vi "example_04_make_installer.vi"() -> ()   [LabVIEW 2015, in "lv-bin-7zip.lvlib" / "v1.lvlib"]
uses:
  v1.lvlib
  <userlib>/antonio-alexander/lv-bin/lv-bin/public/api/v1/advanced/add_data_path_multiple.vi
  advanced/make_installer_exe_simple.vi
  <userlib>/antonio-alexander/lv-bin/lv-bin/public/api/v1/v1.lvlib
  lv-bin-7zip.lvlib
panel:
  out "temp_folder (deleted)":path
  in  "bin_path":path
  out "setup_filename out":path
  out "error out":errorcluster
  in  "setup_filename in":path
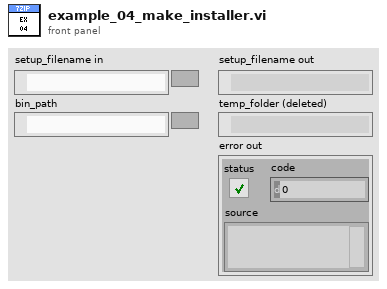
[diagram p1: front panel]
types:
  T1 = enum16{"open", "replace", "create", "open or create", "replace or create", "replace or create with confirmation"}
  T2 = typedef "lv-bin.lvlib/v1.lvlib/temp_dir_config.ctl" = cluster{"root_folder":path, "prefix":string}
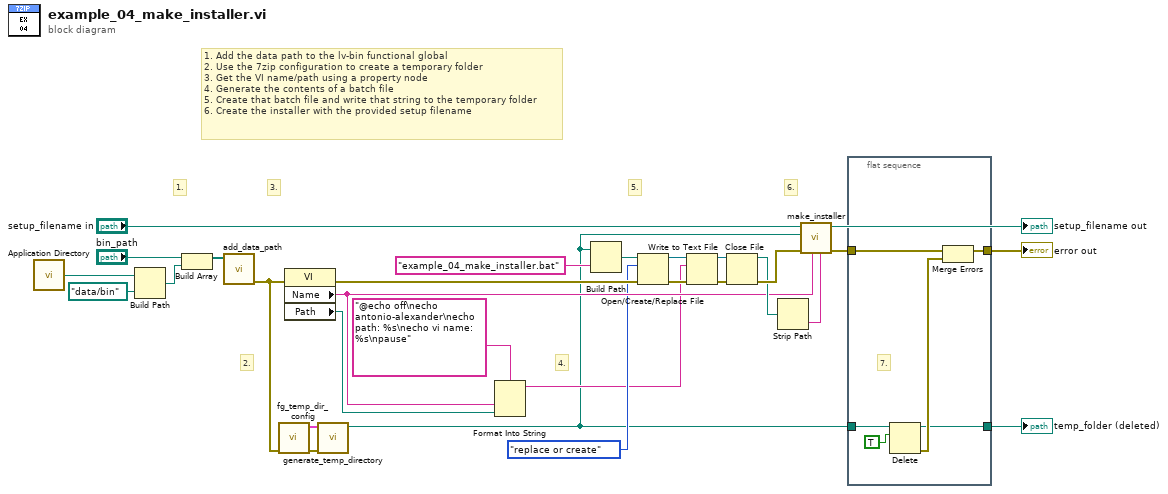
[diagram p0: block diagram]
diagram:
  # "1. Add the data path to the lv-bin functional global\n2. Use the 7zip configuration to create a temporary folder\n3. Get the VI name/path using a property node\n4. Generate the contents of a batch file\n5. Create that batch file and write that string to the temporary folder\n6. Create the installer with the provided setup filename"
  # "4."
  # "3."
  # "6."
  # "5."
  # "2."
  # "1."
  n1 = call <vilib>:"Application Directory.vi"() -> ("Application Directory"=w23:path)
  n2 = Build Path(base path=w23, name or relative path=path "data/bin" ("Application Directory")) -> (appended path=w24:path)
  n3 = Build Array("bin_path", w24) -> (w25:path[])
  n4 = call-poly <userlib>:"add_data_path.vi"("path_to_add []"=w25) -> ("error out"=w16:errorcluster)  [unwired: 10 in]
  n5 = call "fg_temp_dir_config.vi"("error in (no error)"=w16) -> ("error out"=w20:errorcluster, "temp_dir_config out"=w21:T2)  [unwired: 9 in]
  n6 = property class="VI"(error in=w16) -> (error out=w12:errorcluster, "Name"=w14:string, "Path"=w13:path)  [unwired: 1 in, 1 out]
  n7 = call <userlib>:"generate_temp_directory.vi"("error in (no error)"=w20, "configuration"=w21) -> ("temp_dir"=w2:path)  [unwired: 8 in, 1 out]
  n8 = Format Into String(format string="@echo off\necho antonio-alexander\necho path: %s\necho vi name: %s\npause", w14, w13) -> (resulting string=w3:string)  [unwired: 2 in, 1 out]
  n9 = Build Path(base path=w2, name or relative path="example_04_make_installer.bat") -> (appended path=w11:path)
  n10 = Open/Create/Replace File(file path (use dialog)=w11, error in=w12, operation (0:open)=T1."replace or create") -> (refnum out=w8:refnum<file>, error out=w5:errorcluster)  [unwired: 3 in, 1 out]
  n11 = Write to Text File(file (use dialog)=w8, text=w3, error in=w5) -> (refnum out=w7:refnum<file>, error out=w6:errorcluster)  [unwired: 1 in, 1 out]
  n12 = Close File(refnum=w7, error in=w6) -> (path=w15:path, error out=w29:errorcluster)
  n13 = Strip Path(path=w15) -> (name=w17:string)  [unwired: 1 out]
  n14 = call-poly "make_installer.vi"("run_program"=w17, "title"=w14, "error in (no error)"=w29, "installer_directory"=w2, "setup_filename in"="setup_filename in") -> ("error out"=w19:errorcluster, "setup_filename out"=→"setup_filename out":path)  [unwired: 5 in]
  n15 = flat-sequence {
    tunnel: w2 -> [w34]
    tunnel: w19 -> [w32]
    tunnel: [w31] -> w18
    tunnel: [w30] -> w1
    frame #0 {
      # "7."
      n16 = Delete(path (use dialog)=w34, entire hierarchy (F)=TRUE) -> (deleted path=w30:path, error out=w33:errorcluster)  [unwired: 3 in, 1 out]
      n17 = Merge Errors(w32, w33) -> (w31:errorcluster)
    }
  }
  "error out" <- w18
  "temp_folder (deleted)" <- w1
